vi "Configure Histogram1.vi"(5 "Bin Counts (100: 100)":i32(ring)=100 items=["10"=10, "20"=20, "40"=40, "100"=100, "200"=200, "400"=400], 6 "Enable Histogram (F: Disable)":bool, 7 "Auto Histogram Range (T: Enable)":bool=TRUE, 8 "error in (no error)":errorcluster, 9 "Upper Range (0)":dbl, 10 "Lower Range (0)":dbl, 11 "VISA resource name":refnum<visa-resource-name>) -> (0 "error out":errorcluster, 3 "VISA resource name out":refnum<visa-resource-name>)   [LabVIEW 2015, in "Agilent 3446X Series1.lvlib"]
doc: "Configures the settings of histogram."
uses:
  Agilent 3446X Series1.lvlib
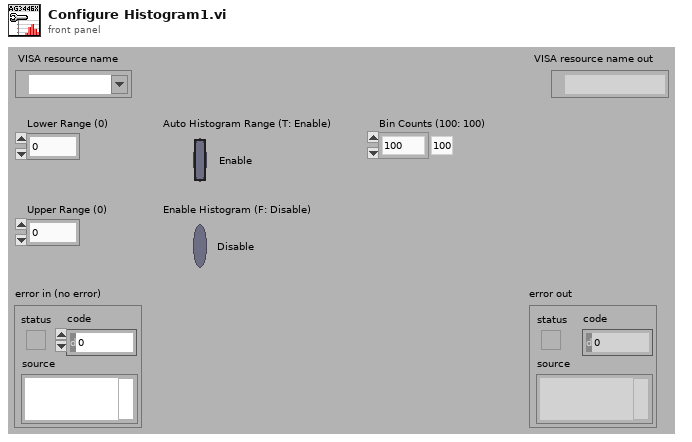
[diagram p1: front panel]
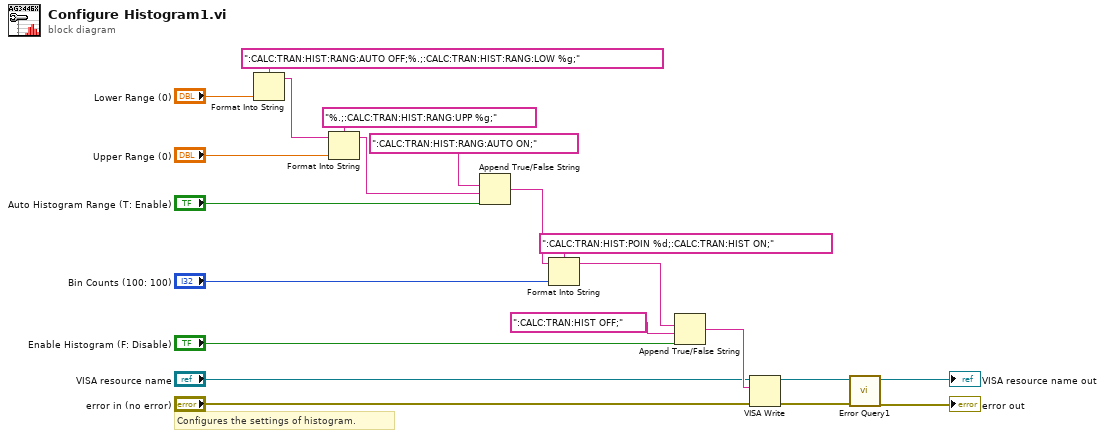
[diagram p0: block diagram]
diagram:
  # "Configures the settings of histogram."
  n1 = Format Into String(format string=":CALC:TRAN:HIST:RANG:AUTO OFF;%.;:CALC:TRAN:HIST:RANG:LOW %g;", "Lower Range (0)") -> (resulting string=w16:string)  [unwired: 2 in, 1 out]
  n2 = Format Into String(format string="%.;:CALC:TRAN:HIST:RANG:UPP %g;", initial string=w16, "Upper Range (0)") -> (resulting string=w1:string)  [unwired: 1 in, 1 out]
  n3 = Append True/False String(1:"Auto Histogram Range (T: Enable)", 2:w1, 3:":CALC:TRAN:HIST:RANG:AUTO ON;") -> (0:w4:string)  [unwired: 1 out]
  n4 = Format Into String(format string=":CALC:TRAN:HIST:POIN %d;:CALC:TRAN:HIST ON;", initial string=w4, "Bin Counts (100: 100)") -> (resulting string=w3:string)  [unwired: 1 in, 1 out]
  n5 = Append True/False String(1:"Enable Histogram (F: Disable)", 2:":CALC:TRAN:HIST OFF;", 3:w3) -> (0:w11:string)  [unwired: 1 out]
  n6 = VISA Write(VISA resource name="VISA resource name", write buffer=w11, error in (no error)="error in (no error)") -> (VISA resource name out=w8:refnum<visa-resource-name>, error out=w7:errorcluster)  [unwired: 1 out]
  n7 = call "Error Query1.vi"("error in (no error)"=w7, "VISA resource name"=w8) -> ("error out"=→"error out":errorcluster, "VISA resource name out"=→"VISA resource name out":refnum<visa-resource-name>)  [unwired: 8 out]
